vi "Set Qualified Names.vi"(10 "Qualified Names":string[](array[string]), 11 "LVLIBP Parser in":refnum<class "LVLIBP Parser.lvclass">) -> (3 "LVLIBP Parser out":refnum<class "LVLIBP Parser.lvclass">)   [LabVIEW 2019, in "LVLIBP CD XML Updater.lvlib" / "LVLIBP Parser.lvclass"]
uses:
  LVLIBP Parser.lvclass
  LVLIBP Parser.lvclass/LVLIBP Parser.ctl
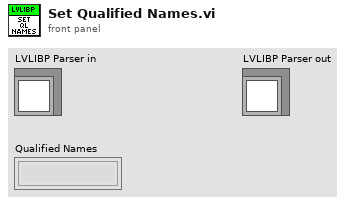
[diagram p1: front panel]
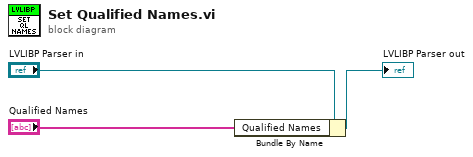
[diagram p0: block diagram]
diagram:
  n1 = Bundle By Name(cluster="LVLIBP Parser in", "Qualified Names"="Qualified Names") -> (→"LVLIBP Parser out":refnum<class "LVLIBP Parser.lvclass">)
